vi "Create from SFTP File.vi"(8 "Error In":errorcluster, 11 "SFTP File In":refnum<class "SFTP File.lvclass">) -> (0 "Error Out":errorcluster, 2 "SFTP Attributes":refnum<class "SFTP Attributes.lvclass">, 3 "SFTP File Out":refnum<class "SFTP File.lvclass">)   [LabVIEW 2018, in "Toolkit.lvlib" / "SFTP Attributes.lvclass"]
uses:
  SFTP Attributes.lvclass
  SFTP File/SFTP File.lvclass
  SFTP File/SFTP File.lvclass/SFTP File.ctl
  SFTP/SFTP.lvclass/SFTP.ctl
  SSH/SSH.lvclass
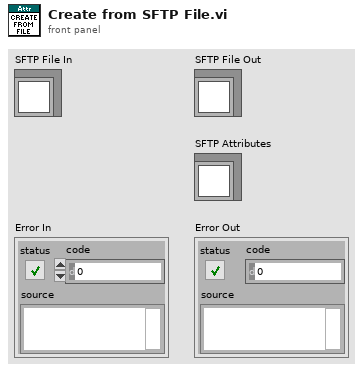
[diagram p1: front panel]
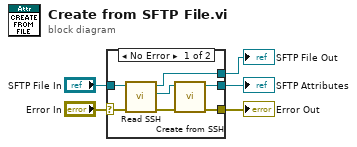
[diagram p0: block diagram]
diagram:
  n1 = case shown="No Error" "Error In" {
    selector: "Error In" -> [w10 w14]
    tunnel: [w11 w14] -> w4
    tunnel: [w12 _] -> w3
    tunnel: "SFTP File In" -> [w9 w13]
    tunnel: [w6 w13] -> w1
    frame No Error {
      n2 = call "Read SSH.vi"("Error In"=w10, "SFTP File In"=w9) -> ("Error Out"=w7:errorcluster, "SSH"=w8:refnum<class "SSH.lvclass">, "SFTP File Out"=w6:refnum<class "SFTP File.lvclass">)  [unwired: 7 in]
      n3 = call "Create from SSH.vi"("Error In"=w7, "SSH"=w8) -> ("Error Out"=w11:errorcluster, "SFTP Attributes"=w12:refnum<class "SFTP Attributes.lvclass">)  [unwired: 8 in]
    }
    frame Error {
    }
  }
  "Error Out" <- w4
  "SFTP Attributes" <- w3
  "SFTP File Out" <- w1
